vi "输入数据解析.vi"(0 "单个参数补充":dbl, 1 "从板号":dbl=1.0, 2 "主板二维码":string="BNET01", 3 "从板二维码":string="BNET01", 5 "主板引用":refnum<vi>, 7 "从板引用":refnum<vi>, 9 "主板选项":string="三级故障阀值", 11 "枚举":enum16{"主板", "从板"}(ring), 12 "快换":bool caption="快换写入") -> (4 "输出数组":dbl[][](array[numeric]), 6 "数组长度":dbl[](array[numeric]), 8 "循环次数":i32, 10 "命令":u32, 14 "名称":string[](array[string]), 15 "命令序号":u32[](array[numeric]))   [LabVIEW 2013] (continued)
                    n4139 = call "输入分辨率计算-EV05.vi"("1字节?"=FALSE, "数值"=w10753, "偏移量"=0.0, "分辨率"=0.001) -> ("低字节"=w10755:dbl, "高字节1"=w10757:dbl)  [unwired: 1 in, 5 out]
                  }
                  frame Enabled {
                    w10760 = 255 ("高字节1")
                  }
                }
                n4140 = Build Array(w10752, w10750) -> (w10751:i32[])
              }
              frame 7 {
                # "单体电压过高"
                n4141 = disable-structure shown="启用" {
                  disable-tunnel: [w10769 w10772] -> w10764
                  disable-tunnel: [w10767 w10772] -> w10762
                  disable-tunnel: w10761 -> [w10766 _]
                  frame Disabled {
                    n4142 = Unbundle By Name(w10766) -> ("单体电压过高"=w10765:dbl)
                    n4143 = call "输入分辨率计算-EV05.vi"("1字节?"=FALSE, "数值"=w10765, "偏移量"=0.0, "分辨率"=0.001) -> ("低字节"=w10767:dbl, "高字节1"=w10769:dbl)  [unwired: 1 in, 5 out]
                  }
                  frame Enabled {
                    w10772 = 255 ("高字节1")
                  }
                }
                n4144 = Build Array(w10764, w10762) -> (w10763:i32[])
              }
              frame 8 {
                # "单体电压过低"
                n4145 = disable-structure shown="启用" {
                  disable-tunnel: [w10781 w10784] -> w10776
                  disable-tunnel: [w10779 w10784] -> w10774
                  disable-tunnel: w10773 -> [w10778 _]
                  frame Disabled {
                    n4146 = Unbundle By Name(w10778) -> ("单体电压过低"=w10777:dbl)
                    n4147 = call "输入分辨率计算-EV05.vi"("1字节?"=FALSE, "数值"=w10777, "偏移量"=0.0, "分辨率"=0.001) -> ("低字节"=w10779:dbl, "高字节1"=w10781:dbl)  [unwired: 1 in, 5 out]
                  }
                  frame Enabled {
                    w10784 = 255 ("高字节1")
                  }
                }
                n4148 = Build Array(w10776, w10774) -> (w10775:i32[])
              }
              frame 9 {
                # "充电电流过高"
                n4149 = disable-structure shown="启用" {
                  disable-tunnel: [w10793 w10796] -> w10788
                  disable-tunnel: [w10791 w10796] -> w10786
                  disable-tunnel: w10785 -> [w10790 _]
                  frame Disabled {
                    n4150 = Unbundle By Name(w10790) -> ("充电电流过高"=w10789:dbl)
                    n4151 = call "输入分辨率计算-EV05.vi"("1字节?"=FALSE, "数值"=w10789, "偏移量"=-3000.0, "分辨率"=0.1) -> ("低字节"=w10791:dbl, "高字节1"=w10793:dbl)  [unwired: 1 in, 5 out]
                  }
                  frame Enabled {
                    w10796 = 255 ("高字节1")
                  }
                }
                n4152 = Build Array(w10788, w10786) -> (w10787:i32[])
              }
              frame 10 {
                # "放电电流过高"
                n4153 = disable-structure shown="启用" {
                  disable-tunnel: [w10805 w10808] -> w10800
                  disable-tunnel: [w10803 w10808] -> w10798
                  disable-tunnel: w10797 -> [w10802 _]
                  frame Disabled {
                    n4154 = Unbundle By Name(w10802) -> ("放电电流过高"=w10801:dbl)
                    n4155 = call "输入分辨率计算-EV05.vi"("1字节?"=FALSE, "数值"=w10801, "偏移量"=-3000.0, "分辨率"=0.1) -> ("低字节"=w10803:dbl, "高字节1"=w10805:dbl)  [unwired: 1 in, 5 out]
                  }
                  frame Enabled {
                    w10808 = 255 ("高字节1")
                  }
                }
                n4156 = Build Array(w10800, w10798) -> (w10799:i32[])
              }
              frame 11 {
                # "单组温度不均衡"
                n4157 = disable-structure shown="启用" {
                  disable-tunnel: [w10815 255 ("高字节1")] -> w10811
                  disable-tunnel: w10809 -> [w10813 _]
                  frame Disabled {
                    n4158 = Unbundle By Name(w10813) -> ("单组温度不均衡"=w10812:dbl)
                    n4159 = call "输入分辨率计算-EV05.vi"("1字节?"=TRUE, "数值"=w10812, "偏移量"=0.0, "分辨率"=1.0) -> ("高字节1"=w10815:dbl)  [unwired: 1 in, 6 out]
                  }
                  frame Enabled {
                  }
                }
                n4160 = Build Array(w10811) -> (w10810:i32[])
              }
              frame 12 {
                # "SOC过高"
                n4161 = Unbundle By Name(w10823) -> ("SOC过高"=w10822:dbl)
                n4162 = call "输入分辨率计算-EV05.vi"("1字节?"=FALSE, "数值"=w10822, "偏移量"=0.0, "分辨率"=0.1) -> ("低字节"=w10824:dbl, "高字节1"=w10825:dbl)  [unwired: 1 in, 5 out]
                n4163 = call "二进制解析-8.6.vi"("索引"=4, "数值"=w10825) -> ("低位子数组"=w10828:i32[])  [unwired: 3 out]
                n4164 = call "二进制解析-8.6.vi"("索引"=4, "数值"=w10824) -> ("低位子数组"=w10820:i32[], "高位子数组"=w10827:i32[])  [unwired: 2 out]
                n4165 = Insert Into Array(array=w10828, new element=w10827) -> (w10826:i32[])  [unwired: 1 in]
                n4166 = call "数值二进制转十进制-8.6.vi"("子数组"=w10826) -> ("十进制数值"=w10821:i32)  [unwired: 4 out]
                n4167 = disable-structure shown="启用" {
                  disable-tunnel: w10821 -> [w10836 _]
                  disable-tunnel: [w10836 255 ("高字节1")] -> w10819
                  disable-tunnel: w10820 -> [w10835 _]
                  disable-tunnel: [w10835 i32[] [] ("低位子数组 29")] -> _
                  frame Disabled {
                  }
                  frame Enabled {
                  }
                }
                n4168 = Build Array(w10819, w10819) -> (w10832:i32[])
              }
              frame 13 {
                # "SOC过低"
                n4169 = Unbundle By Name(w10844) -> ("SOC过低"=w10843:dbl)
                n4170 = call "输入分辨率计算-EV05.vi"("1字节?"=FALSE, "数值"=w10843, "偏移量"=0.0, "分辨率"=0.1) -> ("低字节"=w10841:dbl, "高字节1"=w10842:dbl)  [unwired: 1 in, 5 out]
                n4171 = call "二进制解析-8.6.vi"("索引"=4, "数值"=w10842) -> ("低位子数组"=w10840:i32[])  [unwired: 3 out]
                n4172 = disable-structure shown="启用" {
                  disable-tunnel: w10841 -> [w10852 _]
                  disable-tunnel: [w10852 255 ("高字节1")] -> w10839
                  disable-tunnel: [i32[] [] ("低位子数组 4") _] -> _
                  disable-tunnel: w10840 -> [w10851 _]
                  disable-tunnel: [w10851 i32[] [] ("低位子数组")] -> _
                  frame Disabled {
                  }
                  frame Enabled {
                  }
                }
                n4173 = Build Array(w10839, w10839) -> (w10847:i32[])
              }
              frame 14 {
                # "内阻过大"
                n4174 = disable-structure shown="启用" {
                  disable-tunnel: w10857 -> [w10862 _]
                  disable-tunnel: [w10858 255 ("高字节1")] -> w10855
                  frame Disabled {
                    n4175 = Unbundle By Name(w10862) -> ("内阻过大"=w10861:dbl)
                    n4176 = call "输入分辨率计算-EV05.vi"("1字节?"=TRUE, "数值"=w10861, "分辨率"=0.1) -> ("高字节1"=w10858:dbl)  [unwired: 2 in, 6 out]
                  }
                  frame Enabled {
                  }
                }
                n4177 = Build Array(w10855) -> (w10856:i32[])
              }
              frame 15 {
                # "极柱温度过高"
                n4178 = disable-structure shown="启用" {
                  disable-tunnel: w10866 -> [w10872 _]
                  disable-tunnel: [w10868 255 ("高字节1")] -> w10864
                  frame Disabled {
                    n4179 = Unbundle By Name(w10872) -> ("极柱温度过高"=w10871:dbl)
                    n4180 = call "输入分辨率计算-EV05.vi"("1字节?"=TRUE, "数值"=w10871, "偏移量"=-40.0, "分辨率"=1.0) -> ("高字节1"=w10868:dbl)  [unwired: 1 in, 6 out]
                  }
                  frame Enabled {
                  }
                }
                n4181 = Build Array(w10864) -> (w10865:i32[])
              }
              frame 16 {
                # "SOH过低"
                n4182 = disable-structure shown="启用" {
                  disable-tunnel: [w10879 w10885] -> w10876
                  disable-tunnel: w10875 -> [w10881 _]
                  disable-tunnel: [w10878 w10885] -> w10874
                  frame Enabled {
                    n4183 = Unbundle By Name(w10881) -> ("SOH过低"=w10880:dbl)
                    n4184 = call "输入分辨率计算-EV05.vi"("1字节?"=FALSE, "数值"=w10880, "偏移量"=0.0, "分辨率"=0.1) -> ("低字节"=w10878:dbl, "高字节1"=w10879:dbl)  [unwired: 1 in, 5 out]
                  }
                  frame Disabled {
                    w10885 = 255 ("高字节1")
                  }
                }
                n4185 = Build Array(w10876, w10874) -> (w10877:dbl[])
              }
            }
            n4186 = Insert Into Array(array=w10681, new element=w10682) -> (w10680:dbl[])  [unwired: 1 in]
          }
          n4187 = Build Array(w10677) -> (w10676:dbl[][])
          n4188 = Build Array("一级故障阀值") -> (w10667:string[])
        }
        frame "SOH过低(2)" {
          n4189 = Unbundle By Name(w10891) -> ("一级故障 2"=w10892:refnum<vi>)
          n4190 = property class="Clust (严格)"(reference=w10892) -> ("Value"=w10890:T4)  [unwired: 1 in, 2 out]
          n4191 = for {
            N: 17 -> [_]
            tunnel: w10890 -> [w10902]
            shift-right: [w10899] -> w10896
            shift-left: dbl[] [] -> [w10900]
            i -> [w10903]
            n4192 = case shown="13" w10903 {
              tunnel: w10902 -> [w10904 w10915 w10926 w10936 w10946 w10956 w10968 w10980 w10992 w11004 w11016 w11028 w11042 w11063 w11075 w11084 w11093]
              tunnel: [w10905 w10916 w10927 w10937 w10947 w10958 w10970 w10982 w10994 w11006 w11018 w11029 w11051 w11066 w11074 w11083 w11095] -> w10901
              frame 0, Default {
                # "总电压过高"
                n4193 = disable-structure shown="启用" {
                  disable-tunnel: [w10911 w10914] -> w10907
                  disable-tunnel: [w10910 w10914] -> w10906
                  disable-tunnel: w10904 -> [w10909 _]
                  frame Disabled {
                    n4194 = Unbundle By Name(w10909) -> ("总电压过高"=w10908:dbl)
                    n4195 = call "输入分辨率计算-EV05.vi"("1字节?"=FALSE, "数值"=w10908, "分辨率"=0.1) -> ("低字节"=w10911:dbl, "高字节1"=w10910:dbl)  [unwired: 2 in, 5 out]
                  }
                  frame Enabled {
                    w10914 = 255 ("高字节1")
                  }
                }
                n4196 = Build Array(w10906, w10907) -> (w10905:i32[])
              }
              frame 1 {
                # "总电压过低"
                n4197 = disable-structure shown="启用" {
                  disable-tunnel: [w10922 w10925] -> w10918
                  disable-tunnel: [w10921 w10925] -> w10917
                  disable-tunnel: w10915 -> [w10920 _]
                  frame Disabled {
                    n4198 = Unbundle By Name(w10920) -> ("总电压过低"=w10919:dbl)
                    n4199 = call "输入分辨率计算-EV05.vi"("1字节?"=FALSE, "数值"=w10919, "分辨率"=0.1) -> ("低字节"=w10922:dbl, "高字节1"=w10921:dbl)  [unwired: 2 in, 5 out]
                  }
                  frame Enabled {
                    w10925 = 255 ("高字节1")
                  }
                }
                n4200 = Build Array(w10917, w10918) -> (w10916:i32[])
              }
              frame 2 {
                # "温度过高"
                n4201 = disable-structure shown="启用" {
                  disable-tunnel: [w10932 255 ("高字节1")] -> w10928
                  disable-tunnel: w10926 -> [w10930 _]
                  frame Disabled {
                    n4202 = Unbundle By Name(w10930) -> ("温度过高"=w10929:dbl)
                    n4203 = call "输入分辨率计算-EV05.vi"("1字节?"=TRUE, "数值"=w10929, "偏移量"=-40.0, "分辨率"=1.0) -> ("高字节1"=w10932:dbl)  [unwired: 1 in, 6 out]
                  }
                  frame Enabled {
                  }
                }
                n4204 = Build Array(w10928) -> (w10927:i32[])
              }
              frame 3 {
                # "温度过低"
                n4205 = disable-structure shown="启用" {
                  disable-tunnel: [w10942 255 ("高字节1")] -> w10938
                  disable-tunnel: w10936 -> [w10940 _]
                  frame Disabled {
                    n4206 = Unbundle By Name(w10940) -> ("温度过低"=w10939:dbl)
                    n4207 = call "输入分辨率计算-EV05.vi"("1字节?"=TRUE, "数值"=w10939, "偏移量"=-40.0, "分辨率"=1.0) -> ("高字节1"=w10942:dbl)  [unwired: 1 in, 6 out]
                  }
                  frame Enabled {
                  }
                }
                n4208 = Build Array(w10938) -> (w10937:i32[])
              }
              frame 4 {
                # "整组温度不均衡"
                n4209 = disable-structure shown="启用" {
                  disable-tunnel: [w10952 255 ("高字节1")] -> w10948
                  disable-tunnel: w10946 -> [w10950 _]
                  frame Disabled {
                    n4210 = Unbundle By Name(w10950) -> ("整组温度不均衡"=w10949:dbl)
                    n4211 = call "输入分辨率计算-EV05.vi"("1字节?"=TRUE, "数值"=w10949, "偏移量"=0.0, "分辨率"=1.0) -> ("高字节1"=w10952:dbl)  [unwired: 1 in, 6 out]
                  }
                  frame Enabled {
                  }
                }
                n4212 = Build Array(w10948) -> (w10947:i32[])
              }
              frame 5 {
                # "单组电压不均衡"
                n4213 = disable-structure shown="启用" {
                  disable-tunnel: [w10964 w10967] -> w10959
                  disable-tunnel: [w10962 w10967] -> w10957
                  disable-tunnel: w10956 -> [w10961 _]
                  frame Disabled {
                    n4214 = Unbundle By Name(w10961) -> ("单组电压不均衡"=w10960:dbl)
                    n4215 = call "输入分辨率计算-EV05.vi"("1字节?"=FALSE, "数值"=w10960, "偏移量"=0.0, "分辨率"=0.001) -> ("低字节"=w10962:dbl, "高字节1"=w10964:dbl)  [unwired: 1 in, 5 out]
                  }
                  frame Enabled {
                    w10967 = 255 ("高字节1")
                  }
                }
                n4216 = Build Array(w10959, w10957) -> (w10958:i32[])
              }
              frame 6 {
                # "整组电压不均衡"
                n4217 = disable-structure shown="启用" {
                  disable-tunnel: [w10976 w10979] -> w10971
                  disable-tunnel: [w10974 w10979] -> w10969
                  disable-tunnel: w10968 -> [w10973 _]
                  frame Disabled {
                    n4218 = Unbundle By Name(w10973) -> ("整组电压不均衡"=w10972:dbl)
                    n4219 = call "输入分辨率计算-EV05.vi"("1字节?"=FALSE, "数值"=w10972, "偏移量"=0.0, "分辨率"=0.001) -> ("低字节"=w10974:dbl, "高字节1"=w10976:dbl)  [unwired: 1 in, 5 out]
                  }
                  frame Enabled {
                    w10979 = 255 ("高字节1")
                  }
                }
                n4220 = Build Array(w10971, w10969) -> (w10970:i32[])
              }
              frame 7 {
                # "单体电压过高"
                n4221 = disable-structure shown="启用" {
                  disable-tunnel: [w10988 w10991] -> w10983
                  disable-tunnel: [w10986 w10991] -> w10981
                  disable-tunnel: w10980 -> [w10985 _]
                  frame Disabled {
                    n4222 = Unbundle By Name(w10985) -> ("单体电压过高"=w10984:dbl)
                    n4223 = call "输入分辨率计算-EV05.vi"("1字节?"=FALSE, "数值"=w10984, "偏移量"=0.0, "分辨率"=0.001) -> ("低字节"=w10986:dbl, "高字节1"=w10988:dbl)  [unwired: 1 in, 5 out]
                  }
                  frame Enabled {
                    w10991 = 255 ("高字节1")
                  }
                }
                n4224 = Build Array(w10983, w10981) -> (w10982:i32[])
              }
              frame 8 {
                # "单体电压过低"
                n4225 = disable-structure shown="启用" {
                  disable-tunnel: [w11000 w11003] -> w10995
                  disable-tunnel: [w10998 w11003] -> w10993
                  disable-tunnel: w10992 -> [w10997 _]
                  frame Disabled {
                    n4226 = Unbundle By Name(w10997) -> ("单体电压过低"=w10996:dbl)
                    n4227 = call "输入分辨率计算-EV05.vi"("1字节?"=FALSE, "数值"=w10996, "偏移量"=0.0, "分辨率"=0.001) -> ("低字节"=w10998:dbl, "高字节1"=w11000:dbl)  [unwired: 1 in, 5 out]
                  }
                  frame Enabled {
                    w11003 = 255 ("高字节1")
                  }
                }
                n4228 = Build Array(w10995, w10993) -> (w10994:i32[])
              }
              frame 9 {
                # "充电电流过高"
                n4229 = disable-structure shown="启用" {
                  disable-tunnel: [w11012 w11015] -> w11007
                  disable-tunnel: [w11010 w11015] -> w11005
                  disable-tunnel: w11004 -> [w11009 _]
                  frame Disabled {
                    n4230 = Unbundle By Name(w11009) -> ("充电电流过高"=w11008:dbl)
                    n4231 = call "输入分辨率计算-EV05.vi"("1字节?"=FALSE, "数值"=w11008, "偏移量"=-3000.0, "分辨率"=0.1) -> ("低字节"=w11010:dbl, "高字节1"=w11012:dbl)  [unwired: 1 in, 5 out]
                  }
                  frame Enabled {
                    w11015 = 255 ("高字节1")
                  }
                }
                n4232 = Build Array(w11007, w11005) -> (w11006:i32[])
              }
              frame 10 {
                # "放电电流过高"
                n4233 = disable-structure shown="启用" {
                  disable-tunnel: [w11024 w11027] -> w11019
                  disable-tunnel: [w11022 w11027] -> w11017
                  disable-tunnel: w11016 -> [w11021 _]
                  frame Disabled {
                    n4234 = Unbundle By Name(w11021) -> ("放电电流过高"=w11020:dbl)
                    n4235 = call "输入分辨率计算-EV05.vi"("1字节?"=FALSE, "数值"=w11020, "偏移量"=-3000.0, "分辨率"=0.1) -> ("低字节"=w11022:dbl, "高字节1"=w11024:dbl)  [unwired: 1 in, 5 out]
                  }
                  frame Enabled {
                    w11027 = 255 ("高字节1")
                  }
                }
                n4236 = Build Array(w11019, w11017) -> (w11018:i32[])
              }
              frame 11 {
                # "单组温度不均衡"
                n4237 = disable-structure shown="启用" {
                  disable-tunnel: [w11034 255 ("高字节1")] -> w11030
                  disable-tunnel: w11028 -> [w11032 _]
                  frame Disabled {
                    n4238 = Unbundle By Name(w11032) -> ("单组温度不均衡"=w11031:dbl)
                    n4239 = call "输入分辨率计算-EV05.vi"("1字节?"=TRUE, "数值"=w11031, "偏移量"=0.0, "分辨率"=1.0) -> ("高字节1"=w11034:dbl)  [unwired: 1 in, 6 out]
                  }
                  frame Enabled {
                  }
                }
                n4240 = Build Array(w11030) -> (w11029:i32[])
              }
              frame 12 {
                # "SOC过高"
                n4241 = Unbundle By Name(w11042) -> ("SOC过高"=w11041:dbl)
                n4242 = call "输入分辨率计算-EV05.vi"("1字节?"=FALSE, "数值"=w11041, "偏移量"=0.0, "分辨率"=0.1) -> ("低字节"=w11043:dbl, "高字节1"=w11044:dbl)  [unwired: 1 in, 5 out]
                n4243 = call "二进制解析-8.6.vi"("索引"=4, "数值"=w11044) -> ("低位子数组"=w11047:i32[])  [unwired: 3 out]
                n4244 = call "二进制解析-8.6.vi"("索引"=4, "数值"=w11043) -> ("低位子数组"=w11039:i32[], "高位子数组"=w11046:i32[])  [unwired: 2 out]
                n4245 = Insert Into Array(array=w11047, new element=w11046) -> (w11045:i32[])  [unwired: 1 in]
                n4246 = call "数值二进制转十进制-8.6.vi"("子数组"=w11045) -> ("十进制数值"=w11040:i32)  [unwired: 4 out]
                n4247 = disable-structure shown="启用" {
                  disable-tunnel: w11040 -> [w11055 _]
                  disable-tunnel: [w11055 255 ("高字节1")] -> w11038
                  disable-tunnel: w11039 -> [w11054 _]
                  disable-tunnel: [w11054 i32[] [] ("低位子数组 29")] -> _
                  frame Disabled {
                  }
                  frame Enabled {
                  }
                }
                n4248 = Build Array(w11038, w11038) -> (w11051:i32[])
              }
              frame 13 {
                # "SOC过低"
                n4249 = Unbundle By Name(w11063) -> ("SOC过低"=w11062:dbl)
                n4250 = call "输入分辨率计算-EV05.vi"("1字节?"=FALSE, "数值"=w11062, "偏移量"=0.0, "分辨率"=0.1) -> ("低字节"=w11060:dbl, "高字节1"=w11061:dbl)  [unwired: 1 in, 5 out]
                n4251 = call "二进制解析-8.6.vi"("索引"=4, "数值"=w11061) -> ("低位子数组"=w11059:i32[])  [unwired: 3 out]
                n4252 = disable-structure shown="启用" {
                  disable-tunnel: w11060 -> [w11070 _]
                  disable-tunnel: [w11070 255 ("高字节1")] -> w11058
                  disable-tunnel: w11059 -> [w11069 _]
                  disable-tunnel: [w11069 i32[] [] ("低位子数组")] -> _
                  frame Disabled {
                    (unwired) i32[] [] ("低位子数组 4")
                  }
                  frame Enabled {
                  }
                }
                n4253 = Build Array(w11058, w11058) -> (w11066:i32[])
              }
              frame 14 {
                # "内阻过大"
                n4254 = disable-structure shown="启用" {
                  disable-tunnel: w11075 -> [w11080 _]
                  disable-tunnel: [w11076 255 ("高字节1")] -> w11073
                  frame Disabled {
                    n4255 = Unbundle By Name(w11080) -> ("内阻过大"=w11079:dbl)
                    n4256 = call "输入分辨率计算-EV05.vi"("1字节?"=TRUE, "数值"=w11079, "分辨率"=0.1) -> ("高字节1"=w11076:dbl)  [unwired: 2 in, 6 out]
                  }
                  frame Enabled {
                  }
                }
                n4257 = Build Array(w11073) -> (w11074:i32[])
              }
              frame 15 {
                # "极柱温度过高"
                n4258 = disable-structure shown="启用" {
                  disable-tunnel: w11084 -> [w11090 _]
                  disable-tunnel: [w11086 255 ("高字节1")] -> w11082
                  frame Disabled {
                    n4259 = Unbundle By Name(w11090) -> ("极柱温度过高"=w11089:dbl)
                    n4260 = call "输入分辨率计算-EV05.vi"("1字节?"=TRUE, "数值"=w11089, "偏移量"=-40.0, "分辨率"=1.0) -> ("高字节1"=w11086:dbl)  [unwired: 1 in, 6 out]
                  }
                  frame Enabled {
                  }
                }
                n4261 = Build Array(w11082) -> (w11083:i32[])
              }
              frame 16 {
                # "SOH过低"
                n4262 = disable-structure shown="启用" {
                  disable-tunnel: [w11097 w11103] -> w11094
                  disable-tunnel: w11093 -> [w11099 _]
                  disable-tunnel: [w11096 w11103] -> w11092
                  frame Enabled {
                    n4263 = Unbundle By Name(w11099) -> ("SOH过低"=w11098:dbl)
                    n4264 = call "输入分辨率计算-EV05.vi"("1字节?"=FALSE, "数值"=w11098, "偏移量"=0.0, "分辨率"=0.1) -> ("低字节"=w11096:dbl, "高字节1"=w11097:dbl)  [unwired: 1 in, 5 out]
                  }
                  frame Disabled {
                    w11103 = 255 ("高字节1")
                  }
                }
                n4265 = Build Array(w11094, w11092) -> (w11095:dbl[])
              }
            }
            n4266 = Insert Into Array(array=w10900, new element=w10901) -> (w10899:dbl[])  [unwired: 1 in]
          }
          n4267 = Build Array(w10896) -> (w10895:dbl[][])
          n4268 = Build Array("二级故障阀值") -> (w10886:string[])
        }
        frame "SOH过低(3)" {
          n4269 = Unbundle By Name(w11109) -> ("一级故障 3"=w11110:refnum<vi>)
          n4270 = property class="Clust (严格)"(reference=w11110) -> ("Value"=w11108:T4)  [unwired: 1 in, 2 out]
          n4271 = for {
            N: 17 -> [_]
            tunnel: w11108 -> [w11120]
            shift-right: [w11117] -> w11114
            shift-left: dbl[] [] -> [w11118]
            i -> [w11121]
            n4272 = case shown="16" w11121 {
              tunnel: w11120 -> [w11122 w11133 w11144 w11154 w11164 w11174 w11186 w11198 w11210 w11222 w11234 w11246 w11261 w11282 w11295 w11304 w11313]
              tunnel: [w11123 w11134 w11145 w11155 w11165 w11176 w11188 w11200 w11212 w11224 w11236 w11247 w11270 w11285 w11294 w11303 w11315] -> w11119
              frame 0, Default {
                # "总电压过高"
                n4273 = disable-structure shown="启用" {
                  disable-tunnel: [w11129 w11132] -> w11125
                  disable-tunnel: [w11128 w11132] -> w11124
                  disable-tunnel: w11122 -> [w11127 _]
                  frame Disabled {
                    n4274 = Unbundle By Name(w11127) -> ("总电压过高"=w11126:dbl)
                    n4275 = call "输入分辨率计算-EV05.vi"("1字节?"=FALSE, "数值"=w11126, "分辨率"=0.1) -> ("低字节"=w11129:dbl, "高字节1"=w11128:dbl)  [unwired: 2 in, 5 out]
                  }
                  frame Enabled {
                    w11132 = 255 ("高字节1")
                  }
                }
                n4276 = Build Array(w11124, w11125) -> (w11123:i32[])
              }
              frame 1 {
                # "总电压过低"
                n4277 = disable-structure shown="启用" {
                  disable-tunnel: [w11140 w11143] -> w11136
                  disable-tunnel: [w11139 w11143] -> w11135
                  disable-tunnel: w11133 -> [w11138 _]
                  frame Disabled {
                    n4278 = Unbundle By Name(w11138) -> ("总电压过低"=w11137:dbl)
                    n4279 = call "输入分辨率计算-EV05.vi"("1字节?"=FALSE, "数值"=w11137, "分辨率"=0.1) -> ("低字节"=w11140:dbl, "高字节1"=w11139:dbl)  [unwired: 2 in, 5 out]
                  }
                  frame Enabled {
                    w11143 = 255 ("高字节1")
                  }
                }
                n4280 = Build Array(w11135, w11136) -> (w11134:i32[])
              }
              frame 2 {
                # "温度过高"
                n4281 = disable-structure shown="启用" {
                  disable-tunnel: [w11150 255 ("高字节1")] -> w11146
                  disable-tunnel: w11144 -> [w11148 _]
                  frame Disabled {
                    n4282 = Unbundle By Name(w11148) -> ("温度过高"=w11147:dbl)
                    n4283 = call "输入分辨率计算-EV05.vi"("1字节?"=TRUE, "数值"=w11147, "偏移量"=-40.0, "分辨率"=1.0) -> ("高字节1"=w11150:dbl)  [unwired: 1 in, 6 out]
                  }
                  frame Enabled {
                  }
                }
                n4284 = Build Array(w11146) -> (w11145:i32[])
              }
              frame 3 {
                # "温度过低"
                n4285 = disable-structure shown="启用" {
                  disable-tunnel: [w11160 255 ("高字节1")] -> w11156
                  disable-tunnel: w11154 -> [w11158 _]
                  frame Disabled {
                    n4286 = Unbundle By Name(w11158) -> ("温度过低"=w11157:dbl)
                    n4287 = call "输入分辨率计算-EV05.vi"("1字节?"=TRUE, "数值"=w11157, "偏移量"=-40.0, "分辨率"=1.0) -> ("高字节1"=w11160:dbl)  [unwired: 1 in, 6 out]
                  }
                  frame Enabled {
                  }
                }
                n4288 = Build Array(w11156) -> (w11155:i32[])
              }
              frame 4 {
                # "整组温度不均衡"
                n4289 = disable-structure shown="启用" {
                  disable-tunnel: [w11170 255 ("高字节1")] -> w11166
                  disable-tunnel: w11164 -> [w11168 _]
                  frame Disabled {
                    n4290 = Unbundle By Name(w11168) -> ("整组温度不均衡"=w11167:dbl)
                    n4291 = call "输入分辨率计算-EV05.vi"("1字节?"=TRUE, "数值"=w11167, "偏移量"=0.0, "分辨率"=1.0) -> ("高字节1"=w11170:dbl)  [unwired: 1 in, 6 out]
                  }
                  frame Enabled {
                  }
                }
                n4292 = Build Array(w11166) -> (w11165:i32[])
              }
              frame 5 {
                # "单组电压不均衡"
                n4293 = disable-structure shown="启用" {
                  disable-tunnel: [w11182 w11185] -> w11177
                  disable-tunnel: [w11180 w11185] -> w11175
                  disable-tunnel: w11174 -> [w11179 _]
                  frame Disabled {
                    n4294 = Unbundle By Name(w11179) -> ("单组电压不均衡"=w11178:dbl)
                    n4295 = call "输入分辨率计算-EV05.vi"("1字节?"=FALSE, "数值"=w11178, "偏移量"=0.0, "分辨率"=0.001) -> ("低字节"=w11180:dbl, "高字节1"=w11182:dbl)  [unwired: 1 in, 5 out]
                  }
                  frame Enabled {
                    w11185 = 255 ("高字节1")
                  }
                }
                n4296 = Build Array(w11177, w11175) -> (w11176:i32[])
              }
              frame 6 {
                # "整组电压不均衡"
                n4297 = disable-structure shown="启用" {
                  disable-tunnel: [w11194 w11197] -> w11189
                  disable-tunnel: [w11192 w11197] -> w11187
                  disable-tunnel: w11186 -> [w11191 _]
                  frame Disabled {
                    n4298 = Unbundle By Name(w11191) -> ("整组电压不均衡"=w11190:dbl)
                    n4299 = call "输入分辨率计算-EV05.vi"("1字节?"=FALSE, "数值"=w11190, "偏移量"=0.0, "分辨率"=0.001) -> ("低字节"=w11192:dbl, "高字节1"=w11194:dbl)  [unwired: 1 in, 5 out]
                  }
                  frame Enabled {
                    w11197 = 255 ("高字节1")
                  }
                }
                n4300 = Build Array(w11189, w11187) -> (w11188:i32[])
              }
              frame 7 {
                # "单体电压过高"
                n4301 = disable-structure shown="启用" {
                  disable-tunnel: [w11206 w11209] -> w11201
                  disable-tunnel: [w11204 w11209] -> w11199
                  disable-tunnel: w11198 -> [w11203 _]
                  frame Disabled {
                    n4302 = Unbundle By Name(w11203) -> ("单体电压过高"=w11202:dbl)
                    n4303 = call "输入分辨率计算-EV05.vi"("1字节?"=FALSE, "数值"=w11202, "偏移量"=0.0, "分辨率"=0.001) -> ("低字节"=w11204:dbl, "高字节1"=w11206:dbl)  [unwired: 1 in, 5 out]
                  }
                  frame Enabled {
                    w11209 = 255 ("高字节1")
                  }
                }
                n4304 = Build Array(w11201, w11199) -> (w11200:i32[])
              }
              frame 8 {
                # "单体电压过低"
                n4305 = disable-structure shown="启用" {
                  disable-tunnel: [w11218 w11221] -> w11213
                  disable-tunnel: [w11216 w11221] -> w11211
                  disable-tunnel: w11210 -> [w11215 _]
                  frame Disabled {
                    n4306 = Unbundle By Name(w11215) -> ("单体电压过低"=w11214:dbl)
                    n4307 = call "输入分辨率计算-EV05.vi"("1字节?"=FALSE, "数值"=w11214, "偏移量"=0.0, "分辨率"=0.001) -> ("低字节"=w11216:dbl, "高字节1"=w11218:dbl)  [unwired: 1 in, 5 out]
                  }
                  frame Enabled {
                    w11221 = 255 ("高字节1")
                  }
                }
                n4308 = Build Array(w11213, w11211) -> (w11212:i32[])
              }
              frame 9 {
                # "充电电流过高"
                n4309 = disable-structure shown="启用" {
                  disable-tunnel: [w11230 w11233] -> w11225
                  disable-tunnel: [w11228 w11233] -> w11223
                  disable-tunnel: w11222 -> [w11227 _]
                  frame Disabled {
                    n4310 = Unbundle By Name(w11227) -> ("充电电流过高"=w11226:dbl)
                    n4311 = call "输入分辨率计算-EV05.vi"("1字节?"=FALSE, "数值"=w11226, "偏移量"=-3000.0, "分辨率"=0.1) -> ("低字节"=w11228:dbl, "高字节1"=w11230:dbl)  [unwired: 1 in, 5 out]
                  }
                  frame Enabled {
                    w11233 = 255 ("高字节1")
                  }
                }
                n4312 = Build Array(w11225, w11223) -> (w11224:i32[])
              }
              frame 10 {
                # "放电电流过高"
                n4313 = disable-structure shown="启用" {
                  disable-tunnel: [w11242 w11245] -> w11237
                  disable-tunnel: [w11240 w11245] -> w11235
                  disable-tunnel: w11234 -> [w11239 _]
                  frame Disabled {
                    n4314 = Unbundle By Name(w11239) -> ("放电电流过高"=w11238:dbl)
                    n4315 = call "输入分辨率计算-EV05.vi"("1字节?"=FALSE, "数值"=w11238, "偏移量"=-3000.0, "分辨率"=0.1) -> ("低字节"=w11240:dbl, "高字节1"=w11242:dbl)  [unwired: 1 in, 5 out]
                  }
                  frame Enabled {
                    w11245 = 255 ("高字节1")
                  }
                }
                n4316 = Build Array(w11237, w11235) -> (w11236:i32[])
              }
              frame 11 {
                # "单组温度不均衡"
                n4317 = disable-structure shown="启用" {
                  disable-tunnel: [w11252 255 ("高字节1")] -> w11248
                  disable-tunnel: w11246 -> [w11250 _]
                  frame Disabled {
                    n4318 = Unbundle By Name(w11250) -> ("单组温度不均衡"=w11249:dbl)
                    n4319 = call "输入分辨率计算-EV05.vi"("1字节?"=TRUE, "数值"=w11249, "偏移量"=0.0, "分辨率"=1.0) -> ("高字节1"=w11252:dbl)  [unwired: 1 in, 6 out]
                  }
                  frame Enabled {
                  }
                }
                n4320 = Build Array(w11248) -> (w11247:i32[])
              }
              frame 12 {
                # "SOC过高"
                n4321 = Unbundle By Name(w11261) -> ("SOC过高"=w11260:dbl)
                n4322 = call "输入分辨率计算-EV05.vi"("1字节?"=FALSE, "数值"=w11260, "偏移量"=0.0, "分辨率"=0.1) -> ("低字节"=w11262:dbl, "高字节1"=w11263:dbl)  [unwired: 1 in, 5 out]
                n4323 = call "二进制解析-8.6.vi"("索引"=4, "数值"=w11263) -> ("低位子数组"=w11266:i32[])  [unwired: 3 out]
                n4324 = call "二进制解析-8.6.vi"("索引"=4, "数值"=w11262) -> ("低位子数组"=w11257:i32[], "高位子数组"=w11265:i32[])  [unwired: 2 out]
                n4325 = Insert Into Array(array=w11266, new element=w11265) -> (w11264:i32[])  [unwired: 1 in]
                n4326 = call "数值二进制转十进制-8.6.vi"("子数组"=w11264) -> ("十进制数值"=w11259:i32)  [unwired: 4 out]
                n4327 = disable-structure shown="启用" {
                  disable-tunnel: w11259 -> [w11274 _]
                  disable-tunnel: [w11274 w11275] -> w11258
                  disable-tunnel: w11257 -> [w11273 _]
                  disable-tunnel: [w11273 i32[] [] ("低位子数组 29")] -> _
                  disable-tunnel: [_ w11275] -> w11256
                  frame Disabled {
                  }
                  frame Enabled {
                    w11275 = 255 ("高字节1")
                  }
                }
                n4328 = Build Array(w11258, w11256) -> (w11270:i32[])
              }
              frame 13 {
                # "SOC过低"
                n4329 = Unbundle By Name(w11282) -> ("SOC过低"=w11281:dbl)
                n4330 = call "输入分辨率计算-EV05.vi"("1字节?"=FALSE, "数值"=w11281, "偏移量"=0.0, "分辨率"=0.1) -> ("低字节"=w11279:dbl, "高字节1"=w11280:dbl)  [unwired: 1 in, 5 out]
                n4331 = call "二进制解析-8.6.vi"("索引"=4, "数值"=w11280) -> ("低位子数组"=w11278:i32[])  [unwired: 3 out]
                n4332 = disable-structure shown="启用" {
                  disable-tunnel: w11279 -> [w11290 _]
                  disable-tunnel: [w11290 255 ("高字节1")] -> w11277
                  disable-tunnel: [i32[] [] ("低位子数组 4") _] -> _
                  disable-tunnel: w11278 -> [w11289 _]
                  disable-tunnel: [w11289 i32[] [] ("低位子数组")] -> _
                  frame Disabled {
                  }
                  frame Enabled {
                  }
                }
                n4333 = Build Array(w11277, w11277) -> (w11285:i32[])
              }
              frame 14 {
                # "内阻过大"
                n4334 = disable-structure shown="启用" {
                  disable-tunnel: w11295 -> [w11300 _]
                  disable-tunnel: [w11296 255 ("高字节1")] -> w11293
                  frame Disabled {
                    n4335 = Unbundle By Name(w11300) -> ("内阻过大"=w11299:dbl)
                    n4336 = call "输入分辨率计算-EV05.vi"("1字节?"=TRUE, "数值"=w11299, "分辨率"=0.1) -> ("高字节1"=w11296:dbl)  [unwired: 2 in, 6 out]
                  }
                  frame Enabled {
                  }
                }
                n4337 = Build Array(w11293) -> (w11294:i32[])
              }
              frame 15 {
                # "极柱温度过高"
                n4338 = disable-structure shown="启用" {
                  disable-tunnel: w11304 -> [w11310 _]
                  disable-tunnel: [w11306 255 ("高字节1")] -> w11302
                  frame Disabled {
                    n4339 = Unbundle By Name(w11310) -> ("极柱温度过高"=w11309:dbl)
                    n4340 = call "输入分辨率计算-EV05.vi"("1字节?"=TRUE, "数值"=w11309, "偏移量"=-40.0, "分辨率"=1.0) -> ("高字节1"=w11306:dbl)  [unwired: 1 in, 6 out]
                  }
                  frame Enabled {
                  }
                }
                n4341 = Build Array(w11302) -> (w11303:i32[])
              }
              frame 16 {
                # "SOH过低"
                n4342 = disable-structure shown="启用" {
                  disable-tunnel: [w11317 w11323] -> w11314
                  disable-tunnel: w11313 -> [w11319 _]
                  disable-tunnel: [w11316 w11323] -> w11312
                  frame Enabled {
                    n4343 = Unbundle By Name(w11319) -> ("SOH过低"=w11318:dbl)
                    n4344 = call "输入分辨率计算-EV05.vi"("1字节?"=FALSE, "数值"=w11318, "偏移量"=0.0, "分辨率"=0.1) -> ("低字节"=w11316:dbl, "高字节1"=w11317:dbl)  [unwired: 1 in, 5 out]
                  }
                  frame Disabled {
                    w11323 = 255 ("高字节1")
                  }
                }
                n4345 = Build Array(w11314, w11312) -> (w11315:dbl[])
              }
            }
            n4346 = Insert Into Array(array=w11118, new element=w11119) -> (w11117:dbl[])  [unwired: 1 in]
          }
          n4347 = Build Array(w11114) -> (w11113:dbl[][])
          n4348 = Build Array("三级故障阀值") -> (w11104:string[])
        }
        frame "SOC过高" {
          n4349 = Unbundle By Name(w11329) -> ("一级故障"=w11330:refnum<vi>)
          n4350 = property class="Clust (严格)"(reference=w11330) -> ("Value"=w11328:T4)  [unwired: 1 in, 2 out]
          n4351 = for {
            N: 17 -> [_]
            tunnel: w11328 -> [w11340]
            shift-right: [w11337] -> w11334
            shift-left: dbl[] [] -> [w11338]
            i -> [w11341]
            n4352 = case shown="14" w11341 {
              tunnel: w11340 -> [w11342 w11353 w11364 w11374 w11384 w11394 w11406 w11418 w11430 w11442 w11454 w11466 w11479 w11486 w11498 w11507 w11516]
              tunnel: [w11343 w11354 w11365 w11375 w11385 w11396 w11408 w11420 w11432 w11444 w11456 w11467 w11481 w11487 w11497 w11506 w11518] -> w11339
              frame 0, Default {
                # "总电压过高"
                n4353 = disable-structure shown="启用" {
                  disable-tunnel: [w11349 w11352] -> w11345
                  disable-tunnel: [w11348 w11352] -> w11344
                  disable-tunnel: w11342 -> [w11347 _]
                  frame Disabled {
                    n4354 = Unbundle By Name(w11347) -> ("总电压过高"=w11346:dbl)
                    n4355 = call "输入分辨率计算-EV05.vi"("1字节?"=FALSE, "数值"=w11346, "分辨率"=0.1) -> ("低字节"=w11349:dbl, "高字节1"=w11348:dbl)  [unwired: 2 in, 5 out]
                  }
                  frame Enabled {
                    w11352 = 255 ("高字节1")
                  }
                }
                n4356 = Build Array(w11344, w11345) -> (w11343:i32[])
              }
              frame 1 {
                # "总电压过低"
                n4357 = disable-structure shown="启用" {
                  disable-tunnel: [w11360 w11363] -> w11356
                  disable-tunnel: [w11359 w11363] -> w11355
                  disable-tunnel: w11353 -> [w11358 _]
                  frame Disabled {
                    n4358 = Unbundle By Name(w11358) -> ("总电压过低"=w11357:dbl)
                    n4359 = call "输入分辨率计算-EV05.vi"("1字节?"=FALSE, "数值"=w11357, "分辨率"=0.1) -> ("低字节"=w11360:dbl, "高字节1"=w11359:dbl)  [unwired: 2 in, 5 out]
                  }
                  frame Enabled {
                    w11363 = 255 ("高字节1")
                  }
                }
                n4360 = Build Array(w11355, w11356) -> (w11354:i32[])
              }
              frame 2 {
                # "温度过高"
                n4361 = disable-structure shown="启用" {
                  disable-tunnel: [w11370 255 ("高字节1")] -> w11366
                  disable-tunnel: w11364 -> [w11368 _]
                  frame Disabled {
                    n4362 = Unbundle By Name(w11368) -> ("温度过高"=w11367:dbl)
                    n4363 = call "输入分辨率计算-EV05.vi"("1字节?"=TRUE, "数值"=w11367, "偏移量"=-40.0, "分辨率"=1.0) -> ("高字节1"=w11370:dbl)  [unwired: 1 in, 6 out]
                  }
                  frame Enabled {
                  }
                }
                n4364 = Build Array(w11366) -> (w11365:i32[])
              }
              frame 3 {
                # "温度过低"
                n4365 = disable-structure shown="启用" {
                  disable-tunnel: [w11380 255 ("高字节1")] -> w11376
                  disable-tunnel: w11374 -> [w11378 _]
                  frame Disabled {
                    n4366 = Unbundle By Name(w11378) -> ("温度过低"=w11377:dbl)
                    n4367 = call "输入分辨率计算-EV05.vi"("1字节?"=TRUE, "数值"=w11377, "偏移量"=-40.0, "分辨率"=1.0) -> ("高字节1"=w11380:dbl)  [unwired: 1 in, 6 out]
                  }
                  frame Enabled {
                  }
                }
                n4368 = Build Array(w11376) -> (w11375:i32[])
              }
              frame 4 {
                # "整组温度不均衡"
                n4369 = disable-structure shown="启用" {
                  disable-tunnel: [w11390 255 ("高字节1")] -> w11386
                  disable-tunnel: w11384 -> [w11388 _]
                  frame Disabled {
                    n4370 = Unbundle By Name(w11388) -> ("整组温度不均衡"=w11387:dbl)
                    n4371 = call "输入分辨率计算-EV05.vi"("1字节?"=TRUE, "数值"=w11387, "偏移量"=0.0, "分辨率"=1.0) -> ("高字节1"=w11390:dbl)  [unwired: 1 in, 6 out]
                  }
                  frame Enabled {
                  }
                }
                n4372 = Build Array(w11386) -> (w11385:i32[])
              }
              frame 5 {
                # "单组电压不均衡"
                n4373 = disable-structure shown="启用" {
                  disable-tunnel: [w11402 w11405] -> w11397
                  disable-tunnel: [w11400 w11405] -> w11395
                  disable-tunnel: w11394 -> [w11399 _]
                  frame Disabled {
                    n4374 = Unbundle By Name(w11399) -> ("单组电压不均衡"=w11398:dbl)
                    n4375 = call "输入分辨率计算-EV05.vi"("1字节?"=FALSE, "数值"=w11398, "偏移量"=0.0, "分辨率"=0.001) -> ("低字节"=w11400:dbl, "高字节1"=w11402:dbl)  [unwired: 1 in, 5 out]
                  }
                  frame Enabled {
                    w11405 = 255 ("高字节1")
                  }
                }
                n4376 = Build Array(w11397, w11395) -> (w11396:i32[])
              }
              frame 6 {
                # "整组电压不均衡"
                n4377 = disable-structure shown="启用" {
                  disable-tunnel: [w11414 w11417] -> w11409
                  disable-tunnel: [w11412 w11417] -> w11407
                  disable-tunnel: w11406 -> [w11411 _]
                  frame Disabled {
                    n4378 = Unbundle By Name(w11411) -> ("整组电压不均衡"=w11410:dbl)
                    n4379 = call "输入分辨率计算-EV05.vi"("1字节?"=FALSE, "数值"=w11410, "偏移量"=0.0, "分辨率"=0.001) -> ("低字节"=w11412:dbl, "高字节1"=w11414:dbl)  [unwired: 1 in, 5 out]
                  }
                  frame Enabled {
                    w11417 = 255 ("高字节1")
                  }
                }
                n4380 = Build Array(w11409, w11407) -> (w11408:i32[])
              }
              frame 7 {
                # "单体电压过高"
                n4381 = disable-structure shown="启用" {
                  disable-tunnel: [w11426 w11429] -> w11421
                  disable-tunnel: [w11424 w11429] -> w11419
                  disable-tunnel: w11418 -> [w11423 _]
                  frame Disabled {
                    n4382 = Unbundle By Name(w11423) -> ("单体电压过高"=w11422:dbl)
                    n4383 = call "输入分辨率计算-EV05.vi"("1字节?"=FALSE, "数值"=w11422, "偏移量"=0.0, "分辨率"=0.001) -> ("低字节"=w11424:dbl, "高字节1"=w11426:dbl)  [unwired: 1 in, 5 out]
                  }
                  frame Enabled {
                    w11429 = 255 ("高字节1")
                  }
                }
                n4384 = Build Array(w11421, w11419) -> (w11420:i32[])
              }
              frame 8 {
                # "单体电压过低"
                n4385 = disable-structure shown="启用" {
                  disable-tunnel: [w11438 w11441] -> w11433
                  disable-tunnel: [w11436 w11441] -> w11431
                  disable-tunnel: w11430 -> [w11435 _]
                  frame Disabled {
                    n4386 = Unbundle By Name(w11435) -> ("单体电压过低"=w11434:dbl)
                    n4387 = call "输入分辨率计算-EV05.vi"("1字节?"=FALSE, "数值"=w11434, "偏移量"=0.0, "分辨率"=0.001) -> ("低字节"=w11436:dbl, "高字节1"=w11438:dbl)  [unwired: 1 in, 5 out]
                  }
                  frame Enabled {
                    w11441 = 255 ("高字节1")
                  }
                }
                n4388 = Build Array(w11433, w11431) -> (w11432:i32[])
              }
              frame 9 {
                # "充电电流过高"
                n4389 = disable-structure shown="启用" {
                  disable-tunnel: [w11450 w11453] -> w11445
                  disable-tunnel: [w11448 w11453] -> w11443
                  disable-tunnel: w11442 -> [w11447 _]
                  frame Disabled {
                    n4390 = Unbundle By Name(w11447) -> ("充电电流过高"=w11446:dbl)
                    n4391 = call "输入分辨率计算-EV05.vi"("1字节?"=FALSE, "数值"=w11446, "偏移量"=-3000.0, "分辨率"=0.1) -> ("低字节"=w11448:dbl, "高字节1"=w11450:dbl)  [unwired: 1 in, 5 out]
                  }
                  frame Enabled {
                    w11453 = 255 ("高字节1")
                  }
                }
                n4392 = Build Array(w11445, w11443) -> (w11444:i32[])
              }
              frame 10 {
                # "放电电流过高"
                n4393 = disable-structure shown="启用" {
                  disable-tunnel: [w11462 w11465] -> w11457
                  disable-tunnel: [w11460 w11465] -> w11455
                  disable-tunnel: w11454 -> [w11459 _]
                  frame Disabled {
                    n4394 = Unbundle By Name(w11459) -> ("放电电流过高"=w11458:dbl)
                    n4395 = call "输入分辨率计算-EV05.vi"("1字节?"=FALSE, "数值"=w11458, "偏移量"=-3000.0, "分辨率"=0.1) -> ("低字节"=w11460:dbl, "高字节1"=w11462:dbl)  [unwired: 1 in, 5 out]
                  }
                  frame Enabled {
                    w11465 = 255 ("高字节1")
                  }
                }
                n4396 = Build Array(w11457, w11455) -> (w11456:i32[])
              }
              frame 11 {
                # "单组温度不均衡"
                n4397 = disable-structure shown="启用" {
                  disable-tunnel: [w11472 255 ("高字节1")] -> w11468
                  disable-tunnel: w11466 -> [w11470 _]
                  frame Disabled {
                    n4398 = Unbundle By Name(w11470) -> ("单组温度不均衡"=w11469:dbl)
                    n4399 = call "输入分辨率计算-EV05.vi"("1字节?"=TRUE, "数值"=w11469, "偏移量"=0.0, "分辨率"=1.0) -> ("高字节1"=w11472:dbl)  [unwired: 1 in, 6 out]
                  }
                  frame Enabled {
                  }
                }
                n4400 = Build Array(w11468) -> (w11467:i32[])
              }
              frame 12 {
                # "SOC过高"
                n4401 = Unbundle By Name(w11479) -> ("SOC过高"=w11478:dbl)
                n4402 = call "输入分辨率计算-EV05.vi"("1字节?"=FALSE, "数值"=w11478, "偏移量"=0.0, "分辨率"=0.1) -> ("低字节"=w11476:dbl, "高字节1"=w11477:dbl)  [unwired: 1 in, 5 out]
                n4403 = Build Array(w11477, w11476) -> (w11481:dbl[])
              }
              frame 13 {
                n4404 = disable-structure shown="启用" {
                  disable-tunnel: w11486 -> [w11491 _]
                  disable-tunnel: [w11489 w11495] -> w11485
                  disable-tunnel: [w11488 w11495] -> w11484
                  frame Disabled {
                    n4405 = Unbundle By Name(w11491) -> ("SOC过低"=w11490:dbl)
                    n4406 = call "输入分辨率计算-EV05.vi"("1字节?"=FALSE, "数值"=w11490, "偏移量"=0.0, "分辨率"=0.1) -> ("低字节"=w11488:dbl, "高字节1"=w11489:dbl)  [unwired: 1 in, 5 out]
                  }
                  frame Enabled {
                    w11495 = 255 ("高字节1")
                  }
                }
                n4407 = Build Array(w11485, w11484) -> (w11487:i32[])
              }
              frame 14 {
                # "内阻过大"
                n4408 = disable-structure shown="启用" {
                  disable-tunnel: w11498 -> [w11503 _]
                  disable-tunnel: [w11499 255 ("高字节1")] -> w11496
                  frame Disabled {
                    n4409 = Unbundle By Name(w11503) -> ("内阻过大"=w11502:dbl)
                    n4410 = call "输入分辨率计算-EV05.vi"("1字节?"=TRUE, "数值"=w11502, "分辨率"=0.1) -> ("高字节1"=w11499:dbl)  [unwired: 2 in, 6 out]
                  }
                  frame Enabled {
                  }
                }
                n4411 = Build Array(w11496) -> (w11497:i32[])
              }
              frame 15 {
                # "极柱温度过高"
                n4412 = disable-structure shown="启用" {
                  disable-tunnel: w11507 -> [w11513 _]
                  disable-tunnel: [w11509 255 ("高字节1")] -> w11505
                  frame Disabled {
                    n4413 = Unbundle By Name(w11513) -> ("极柱温度过高"=w11512:dbl)
                    n4414 = call "输入分辨率计算-EV05.vi"("1字节?"=TRUE, "数值"=w11512, "偏移量"=-40.0, "分辨率"=1.0) -> ("高字节1"=w11509:dbl)  [unwired: 1 in, 6 out]
                  }
                  frame Enabled {
                  }
                }
                n4415 = Build Array(w11505) -> (w11506:i32[])
              }
              frame 16 {
                # "SOH过低"
                n4416 = disable-structure shown="启用" {
                  disable-tunnel: [w11530 w11538] -> w11517
                  disable-tunnel: w11516 -> [w11527 _]
                  disable-tunnel: [w11519 w11538] -> w11515
                  frame Disabled {
                    n4417 = Unbundle By Name(w11527) -> ("SOH过低"=w11526:dbl)
                    n4418 = call "输入分辨率计算-EV05.vi"("1字节?"=FALSE, "数值"=w11526, "偏移量"=0.0, "分辨率"=0.1) -> ("低字节"=w11528:dbl, "高字节1"=w11529:dbl)  [unwired: 1 in, 5 out]
                    n4419 = call "二进制解析-8.6.vi"("索引"=4, "数值"=w11529) -> ("低位子数组"=w11532:i32[])  [unwired: 3 out]
                    n4420 = call "二进制解析-8.6.vi"("索引"=4, "数值"=w11528) -> ("低位子数组"=w11521:i32[], "高位子数组"=w11531:i32[])  [unwired: 2 out]
                    n4421 = call "二进制解析-8.6.vi"("索引"=4, "数值"=0) -> ("低位子数组"=w11522:i32[])  [unwired: 3 out]
                    n4422 = Insert Into Array(array=w11532, new element=w11531) -> (w11525:i32[])  [unwired: 1 in]
                    n4423 = Insert Into Array(array=w11521, new element=w11522) -> (w11520:i32[])  [unwired: 1 in]
                    n4424 = call "数值二进制转十进制-8.6.vi"("子数组"=w11525) -> ("十进制数值"=w11530:i32)  [unwired: 4 out]
                    n4425 = call "数值二进制转十进制-8.6.vi"("子数组"=w11520) -> ("十进制数值"=w11519:i32)  [unwired: 4 out]
                  }
                  frame Enabled {
                    w11538 = 255 ("高字节1")
                  }
                }
                n4426 = Build Array(w11517, w11515) -> (w11518:i32[])
              }
            }
            n4427 = Insert Into Array(array=w11338, new element=w11339) -> (w11337:dbl[])  [unwired: 1 in]
          }
          n4428 = Build Array(w11334) -> (w11333:dbl[][])
          n4429 = Build Array("一级故障阀值") -> (w11324:string[])
        }
        frame "SOC过高(2)" {
          n4430 = Unbundle By Name(w11544) -> ("一级故障 2"=w11545:refnum<vi>)
          n4431 = property class="Clust (严格)"(reference=w11545) -> ("Value"=w11543:T4)  [unwired: 1 in, 2 out]
          n4432 = for {
            N: 17 -> [_]
            tunnel: w11543 -> [w11555]
            shift-right: [w11552] -> w11549
            shift-left: dbl[] [] -> [w11553]
            i -> [w11556]
            n4433 = case shown="12" w11556 {
              tunnel: w11555 -> [w11557 w11568 w11579 w11589 w11599 w11609 w11621 w11633 w11645 w11657 w11669 w11681 w11694 w11701 w11713 w11722 w11731]
              tunnel: [w11558 w11569 w11580 w11590 w11600 w11611 w11623 w11635 w11647 w11659 w11671 w11682 w11696 w11702 w11712 w11721 w11733] -> w11554
              frame 0, Default {
                # "总电压过高"
                n4434 = disable-structure shown="启用" {
                  disable-tunnel: [w11564 w11567] -> w11560
                  disable-tunnel: [w11563 w11567] -> w11559
                  disable-tunnel: w11557 -> [w11562 _]
                  frame Disabled {
                    n4435 = Unbundle By Name(w11562) -> ("总电压过高"=w11561:dbl)
                    n4436 = call "输入分辨率计算-EV05.vi"("1字节?"=FALSE, "数值"=w11561, "分辨率"=0.1) -> ("低字节"=w11564:dbl, "高字节1"=w11563:dbl)  [unwired: 2 in, 5 out]
                  }
                  frame Enabled {
                    w11567 = 255 ("高字节1")
                  }
                }
                n4437 = Build Array(w11559, w11560) -> (w11558:i32[])
              }
              frame 1 {
                # "总电压过低"
                n4438 = disable-structure shown="启用" {
                  disable-tunnel: [w11575 w11578] -> w11571
                  disable-tunnel: [w11574 w11578] -> w11570
                  disable-tunnel: w11568 -> [w11573 _]
                  frame Disabled {
